vi "Graph.vi"(11 "Notifier in":refnum<notifier>) -> ()   [LabVIEW 2024]
panel:
  out "Current Array":T1(array[cluster])
  out "Voltage Array":T1(array[cluster])
  out "Current & Voltage Graph":waveform(dbl)[](graph)
  # "These controls have associated \"Value Changed\" events configured in the Event Structure on the diagram.\n\nReplace them (and reconfigure the Event Structure) with the controls you need for your application. \n\nOther processes communicate with this Module via its Public API (wrappers for its Request Events).\n\nThis Module communicates with other processes via its Broadcast Events.\nAny process that wants to receive these messages can register for this module's Broadcast events."
  # "This template is for the DQMH framework. See the block diagram for more information on how to use this template."
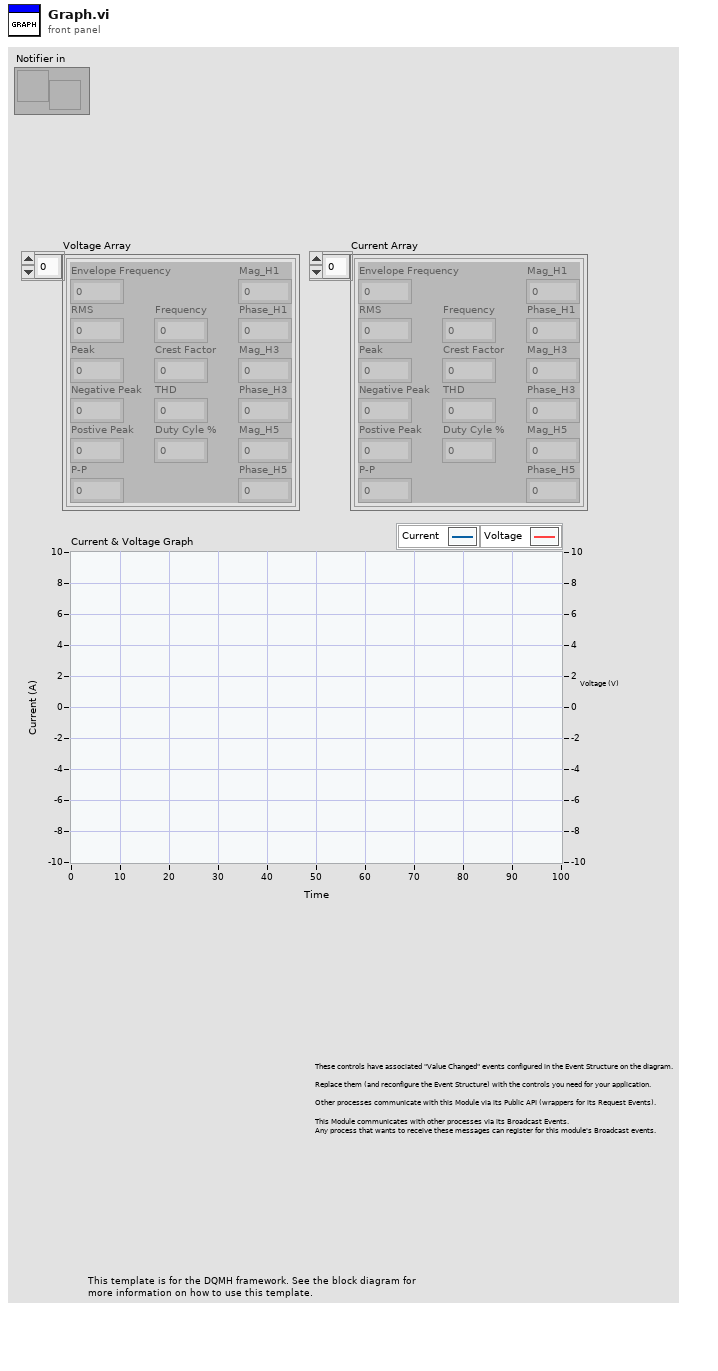
[diagram p1: front panel]
types:
  T1 = cluster{"RMS":dbl, "Envelope Frequency":dbl, "Peak":dbl, "Crest Factor":dbl, "Duty Cyle %":dbl, "P-P":dbl, "Frequency":dbl, "THD":dbl, "Postive Peak":dbl, "Negative Peak":dbl, "Mag_H1":dbl, "Phase_H1":dbl, "Mag_H3":dbl, "Phase_H3":dbl, "Mag_H5":dbl, "Phase_H5":dbl}[]
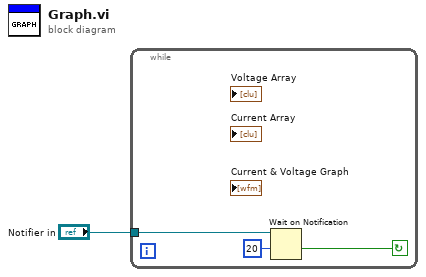
[diagram p0: block diagram]
diagram:
  n1 = while {
    tunnel: "Notifier in" -> [w3]
    stop <- w2 continue-if-true
    n2 = Wait on Notification(notifier=w3, timeout in ms (-1)=20) -> (timed out?=w2:bool)  [unwired: 2 in, 3 out]
  }
